vi "sample-code.vi"() -> ()   [LabVIEW 2016]
uses:
  Pressure-Transducer_class/Pressure-Transducer.lvclass
  S:/Dcar/National_Instruments/LabView-2016/Practice/Goop-Class/Modbus-Instr_class/Modbus-Instr.lvclass
  Modbus-Instr_class/Modbus-Instr.lvclass
panel:
  out "Data":dbl[](array[numeric])
  in  "Modbus-Reg":u16[](array[numeric])
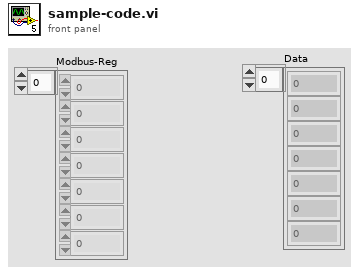
[diagram p1: front panel]
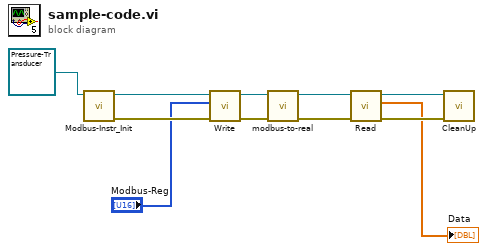
[diagram p0: block diagram]
diagram:
  n1 = call "Modbus-Instr_Init.vi"("object in"=refnum<class "Pressure-Transducer.lvclass"> refnum ("Modbus-Instr")) -> ("error out"=w10:errorcluster, "object out"=w11:refnum<class "Pressure-Transducer.lvclass">)  [unwired: 9 in]
  n2 = call-dynamic "Write.vi"("error in (no error)"=w10, "Modbus-Reg"="Modbus-Reg", "object in"=w11) -> ("error out"=w7:errorcluster, "object out"=w9:refnum<class "Pressure-Transducer.lvclass">)  [unwired: 7 in]
  n3 = call-dynamic "modbus-to-real.vi"("error in (no error)"=w7, "object in"=w9) -> ("error out"=w4:errorcluster, "object out"=w6:refnum<class "Pressure-Transducer.lvclass">)  [unwired: 8 in]
  n4 = call-dynamic "Read.vi"("error in (no error)"=w4, "object in"=w6) -> ("error out"=w3:errorcluster, "Data"=→"Data":dbl[], "object out"=w5:refnum<class "Pressure-Transducer.lvclass">)  [unwired: 7 in]
  n5 = call-dynamic "CleanUp.vi"("error in (no error)"=w3, "object in"=w5) -> ()  [unwired: 8 in, 2 out]
